vi "DQ_transforming.vi"(2 "DQ":cluster{"q":T1, "qe":T1}, 3 "Vector":cluster{"q":T1, "qe":T1}={"q"=[1.0, 0.0, 0.0, 0.0], "qe"=[]}) -> (0 "transformedVector":T1=[1.0, 0.0, 0.0, 0.0], 1 "transformedVector":cluster{"q":T1, "qe":T1})   [LabVIEW 2014]
doc: "单位四元数实现图片旋转"
uses:
  <vilib>/robotics/Kinematics/Quaternion.ctl
  <vilib>/robotics/Kinematics/NI_Kinematics.lvlib
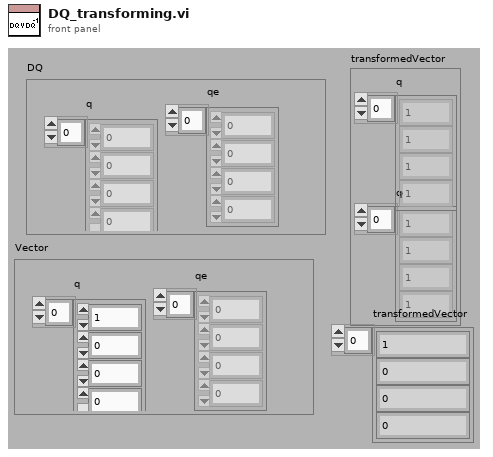
[diagram p1: front panel]
types:
  T1 = typedef "NI_Kinematics.lvlib/Quaternion.ctl" = dbl[]
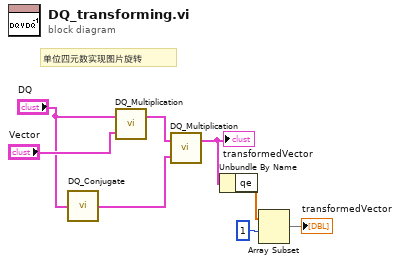
[diagram p0: block diagram]
diagram:
  # "单位四元数实现图片旋转"
  n1 = call "DQ_Conjugate.vi"("DQ2"="DQ") -> ("Conjugate"=w1:cluster{"q":T1, "qe":T1})
  n2 = call "DQ_Multiplication.vi"("DQ2"="Vector", "DQ1"="DQ") -> ("Product"=w7:cluster{"q":T1, "qe":T1})  [unwired: 1 in]
  n3 = call "DQ_Multiplication.vi"("DQ2"=w1, "DQ1"=w7) -> ("Product"=w5:cluster{"q":T1, "qe":T1})  [unwired: 1 in]
  "transformedVector" <- w5
  n4 = Unbundle By Name(w5) -> ("qe"=w4:T1)
  n5 = Array Subset(array=w4, index=1 ("索引")) -> (→"transformedVector":T1)  [unwired: 1 in]
